vi "WPI_UtilitiesFRC SendMessageToConsole.vi"(0 "Message":string, 11 "error in (no error)":errorcluster) -> (15 "error out":errorcluster)   [LabVIEW 2025]
doc: "Appends the string message to the console and DS log..\n\nThis software is licensed. Open the labview\\readme\\WPI Robotics Library Open Source License.txt file for more information."
uses:
  FRC_NetworkTablesLV.dll
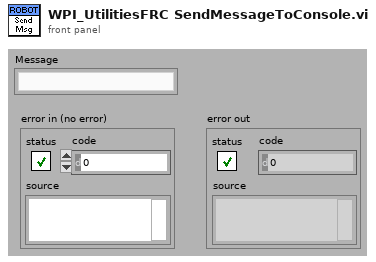
[diagram p1: front panel]
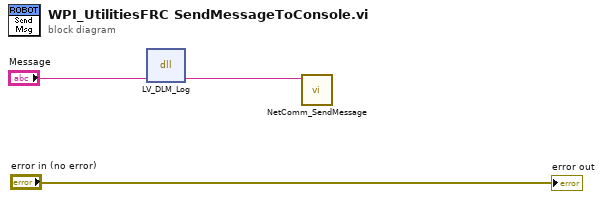
[diagram p0: block diagram]
diagram:
  n1 = dll-call lib="FRC_NetworkTablesLV.*" fn="LV_DLM_Log"("message"="Message") -> ("message"=w1:string)  [unwired: 4 in, 2 out]
  n2 = call <vilib>:"NetComm_SendMessage.vi"("Message"=w1) -> ()  [unwired: 11 in]
  "error out" <- "error in (no error)"
